vi "_UpdateCalTable.vi"(6 "CalResultIn":T1, 7 "Valid Peak?":bool, 8 "Calibration":dbl[][](array[numeric])=[[0.0, 0.0], [59.06, 8007.972231628852], [175.13, 24051.118700948115], [609.3, 84085.25564675158], [616.46, 85075.93195639057], [906.67, 125230.14589777726], [1254.9, 173425.601618889], [1487.09, 205562.74183429], [1500.0, 207349.59949474406]] format="%.2f", 9 "RefMass":dbl, 10 "MassFound":dbl, 11 "Found":bool) -> (0 "CalibrationOut":dbl[][](array[numeric])=[[0.0, 0.0], [59.06, 8007.972231628852], [175.13, 24051.118700948115], [609.3, 84085.25564675158], [616.46, 85075.93195639057], [906.67, 125230.14589777726], [1254.9, 173425.601618889], [1487.09, 205562.74183429], [1500.0, 207349.59949474406]] format="%.2f", 1 "CalValid":bool, 2 "CalOK":bool, 3 "CalResultOut":T1, 4 "New DAC":dbl, 5 "ClosestIndex":i32)   [LabVIEW 2015]
uses:
  Type/_CalibrationResult.ctl
  Type/_Log Command.ctl
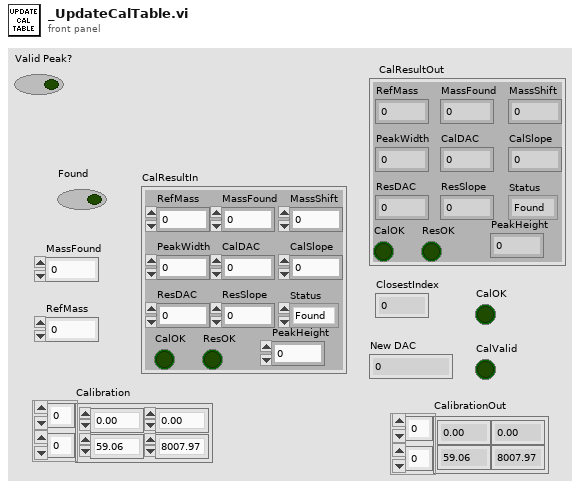
[diagram p1: front panel]
types:
  T1 = typedef "_CalibrationResult.ctl" = cluster{"RefMass":dbl, "MassFound":dbl, "MassShift":dbl, "PeakWidth":dbl, "CalDAC":dbl, "CalSlope":dbl, "ResDAC":dbl, "ResSlope":dbl, "Status":enum16{"Found", "Missing", "Not Used"}, "CalOK":bool, "ResOK":bool, "PeakHeight":dbl}
  T2 = typedef "_Log Command.ctl" = enum16{"No Command", "Open", "Read", "Write", "Close", "Check Size"}
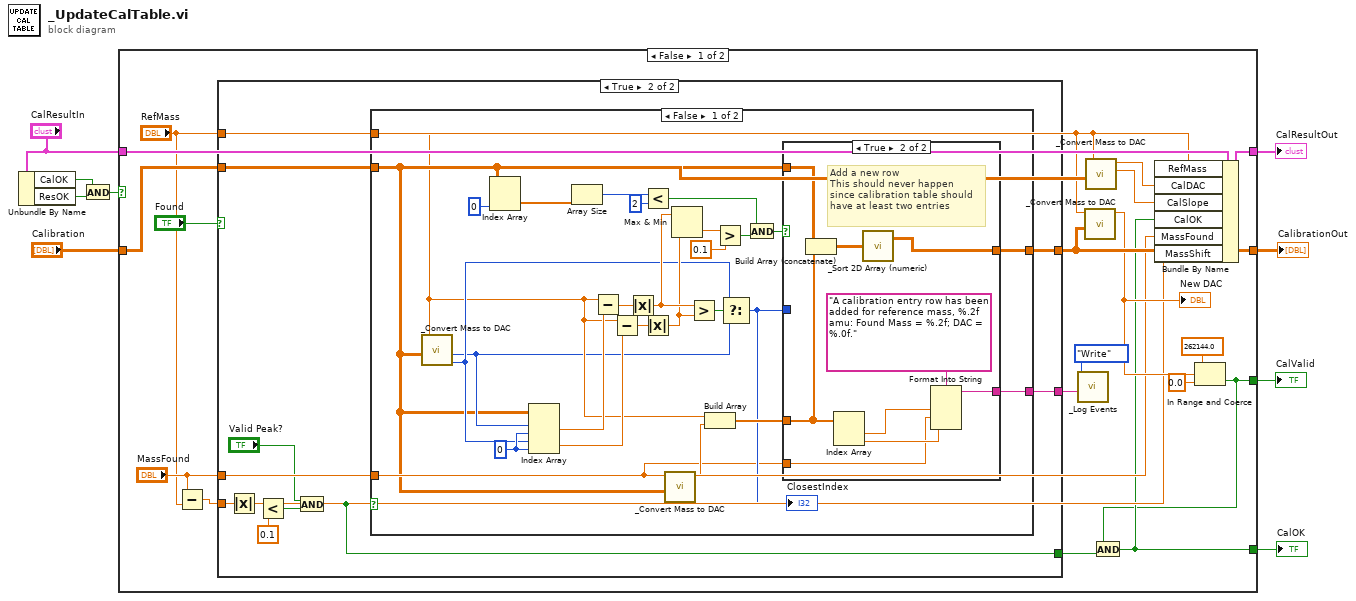
[diagram p0: block diagram]
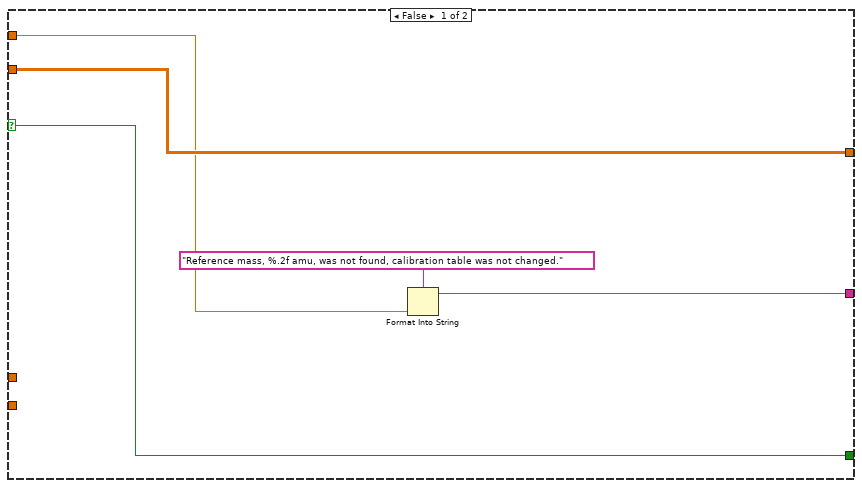
[diagram p2: hidden frame]
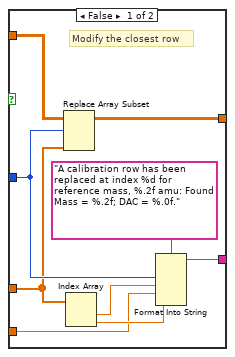
[diagram p3: hidden frame]
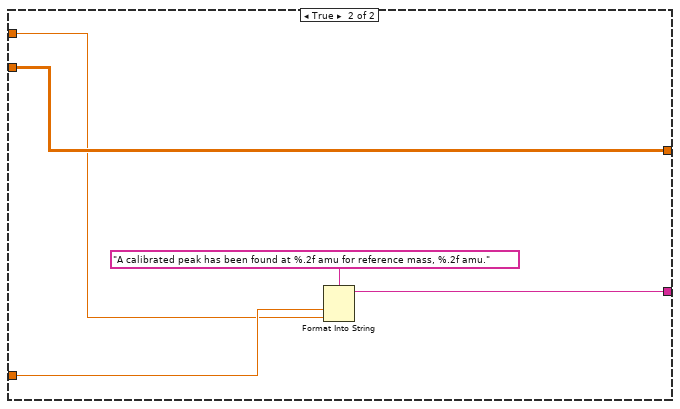
[diagram p4: hidden frame]
diagram:
  n1 = Unbundle By Name("CalResultIn") -> ("CalOK"=w2:bool, "ResOK"=w1:bool)
  n2 = And(x=w2, y=w1) -> (x .and. y?=w3:bool)
  n3 = case shown="False" w3 {
    selector: w3 -> [_ w94]
    tunnel: [w18 w96] -> w8
    tunnel: "CalResultIn" -> [w19 w96]
    tunnel: [w24 w95] -> w7
    tunnel: "Calibration" -> [w23 w95]
    tunnel: [w12 w94] -> w5
    tunnel: [w11 w94] -> w4
    frame False {
      n4 = Subtract(x="MassFound", y="RefMass") -> (x-y=w13:dbl)
      n5 = case shown="True" "Found" {
        selector: "Found" -> [w28 _]
        tunnel: [w32 w43] -> w24
        tunnel: "RefMass" -> [w30 w42]
        tunnel: w23 -> [w32 w41]
        tunnel: [w29 w40] -> w26
        tunnel: "MassFound" -> [_ w39]
        tunnel: w13 -> [_ w36]
        tunnel: [w28 w34] -> w10
        frame False {
          n6 = Format Into String(format string="Reference mass, %.2f amu, was not found, calibration table was not changed.", w30) -> (resulting string=w29:string)  [unwired: 2 in, 1 out]
        }
        frame True {
          n7 = Absolute Value(x=w36) -> (abs(x)=w38:dbl)
          n8 = Less?(x=w38, y=0.1) -> (x < y?=w35:bool)
          n9 = And(x="Valid Peak?", y=w35) -> (x .and. y?=w34:bool)
          n10 = case shown="False" w34 {
            tunnel: [w51 w93] -> w43
            tunnel: w42 -> [w50 w90]
            tunnel: w41 -> [w46 w93]
            tunnel: w39 -> [w47 w91]
            tunnel: [w49 w89] -> w40
            frame False {
              w70 = 0 ("disabled index (col)")
              n11 = call "_Convert Mass to DAC.vi"("Calibration Table"=w46, "Mass"=w50) -> ("LowerIndex"=w55:i32, "UpperIndex"=w48:i32)  [unwired: 2 in, 2 out]
              n12 = Index Array(array=w46, index (col)=0 ("disabled index (col)")) -> (element=w44:dbl[])  [unwired: 1 in]
              n13 = Index Array(array=w46, index (row) #1=w48, index (col) #1=w70, index (row) #2=w55, index (col) #2=w70) -> (element #1=w69:dbl, element #2=w68:dbl)
              n14 = Array Size(array=w44) -> (size(s)=w60:i32)
              n15 = Subtract(x=w50, y=w69) -> (x-y=w67:dbl)
              n16 = Subtract(x=w50, y=w68) -> (x-y=w66:dbl)
              n17 = Absolute Value(x=w67) -> (abs(x)=w64:dbl)
              n18 = Less?(x=w60, y=2) -> (x < y?=w57:bool)
              n19 = Absolute Value(x=w66) -> (abs(x)=w63:dbl)
              n20 = call "_Convert Mass to DAC.vi"("Calibration Table"=w46, "Mass"=w47) -> ("DAC Value"=w54:dbl)  [unwired: 2 in, 3 out]
              n21 = Max & Min(x=w64, y=w63) -> (min(x,y)=w62:dbl)  [unwired: 1 out]
              n22 = Greater?(x=w64, y=w63) -> (0:w65:bool)
              n23 = Build Array(w50, w54) -> (w53:dbl[])
              n24 = Greater?(x=w62, y=0.1) -> (0:w58:bool)
              n25 = Select(t=w55, s=w65, f=w48) -> (s? t:f=w52:i32)
              "ClosestIndex" <- w52
              n26 = And(x=w57, y=w58) -> (x .and. y?=w56:bool)
              n27 = case shown="True" w56 {
                tunnel: w46 -> [w79 w83]
                tunnel: w53 -> [w74 w82]
                tunnel: w52 -> [w76 _]
                tunnel: [w73 w80] -> w51
                tunnel: [w75 w86] -> w49
                tunnel: w47 -> [w71 w84]
                frame False {
                  # "Modify the closest row"
                  n28 = Replace Array Subset(array=w79, new element=w74, index (row)=w76) -> (w73:dbl[][])  [unwired: 1 in]
                  n29 = Index Array(array=w74) -> (element #1=w78:dbl, element #2=w72:dbl)  [unwired: 2 in]
                  n30 = Format Into String(format string="A calibration row has been replaced at index %d for reference mass, %.2f amu: Found Mass = %.2f; DAC = %.0f.", w76, w78, w71, w72) -> (resulting string=w75:string)  [unwired: 2 in, 1 out]
                }
                frame True {
                  # "Add a new row\nThis should never happen\nsince calibration table should\nhave at least two entries"
                  n31 = Build Array (concatenate)(w83, w82) -> (w81:dbl[][])
                  n32 = Index Array(array=w82) -> (element #1=w88:dbl, element #2=w85:dbl)  [unwired: 2 in]
                  n33 = call "_Sort 2D Array (numeric).vi"("Unsorted 2D Array"=w81) -> ("Sorted 2D Array"=w80:dbl[][])  [unwired: 4 in, 1 out]
                  n34 = Format Into String(format string="A calibration entry row has been added for reference mass, %.2f amu: Found Mass = %.2f; DAC = %.0f.", w88, w84, w85) -> (resulting string=w86:string)  [unwired: 2 in, 1 out]
                }
              }
            }
            frame True {
              n35 = Format Into String(format string="A calibrated peak has been found at %.2f amu for reference mass, %.2f amu.", w91, w90) -> (resulting string=w89:string)  [unwired: 2 in, 1 out]
            }
          }
        }
      }
      n36 = call "_Log Events.vi"("Event"=w26, "Log Command"=_Log_Command."Write") -> ()  [unwired: 6 in, 2 out]
      n37 = call "_Convert Mass to DAC.vi"("Calibration Table"=w24, "Mass"="RefMass") -> ("DAC Value"=w20:dbl)  [unwired: 2 in, 3 out]
      "New DAC" <- w20
      n38 = call "_Convert Mass to DAC.vi"("Calibration Table"=w23, "Mass"="RefMass") -> ("Slope"=w17:dbl, "DAC Value"=w16:dbl)  [unwired: 2 in, 2 out]
      n39 = In Range and Coerce(upper limit=262144.0, x=w20, lower limit=0.0) -> (In Range?=w11:bool)  [unwired: 1 out]
      n40 = And(x=w11, y=w10) -> (x .and. y?=w12:bool)
      n41 = Bundle By Name(cluster=w19, "RefMass"="RefMass", "CalDAC"=w16, "CalSlope"=w17, "CalOK"=w12, "MassFound"="MassFound", "MassShift"=w13) -> (w18:T1)
    }
    frame True {
      # "The given reference peak has met all calibration criteria from the previous iteration.\nNo further adjustment required."
    }
  }
  "CalResultOut" <- w8
  "CalibrationOut" <- w7
  "CalOK" <- w5
  "CalValid" <- w4
